vi "Nabız Ölçer.vi"() -> ()   [LabVIEW 2017]
uses:
  <vilib>/MakerHub/LINX/Public/Peripherals/Analog/Analog Read 1 Chan.vi
  <vilib>/MakerHub/LINX/Public/Peripherals/Analog/Analog Read N Chans.vi
  <vilib>/MakerHub/LINX/Private/Local IO/LinxAnalogRead.vi
  <vilib>/MakerHub/LINX/Public/Utilities/Check Channel.vi
  <vilib>/MakerHub/LINX/Public/Utilities/Open Serial.vi
  <vilib>/MakerHub/LINX/Private/Utilties/Generate Error.vi
  <vilib>/MakerHub/LINX/LMH-LINX.lvlib
panel:
  in  "Serial Port":refnum<visa-resource-name>="N/A"
  in  "Analog Channel":u8
  out "Waveform Chart":dbl(graph)
  in  "Stop":bool
  out "nabız":dbl
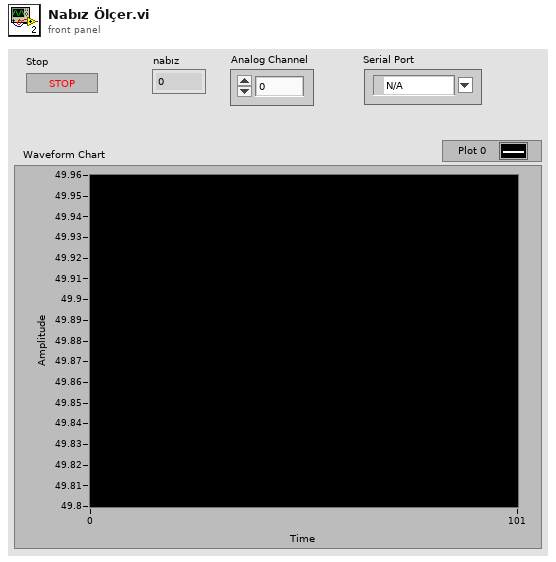
[diagram p1: front panel]
types:
  T1 = enum16{"open", "replace", "create", "open or create", "replace or create", "replace or create with confirmation"}
  T2 = typedef "LMH-LINX.lvlib/LINX Ref.ctl" = cluster{"IO":T3, "Interface":T4, "LINX Device Config":T5}
  T3 = typedef "LMH-LINX.lvlib/Platform.ctl" = enum16{"Remote", "Local"}
  T4 = typedef "LMH-LINX.lvlib/Interface.ctl" = enum16{"Serial", "TCP"}
  T5 = typedef "LMH-LINX.lvlib/Device.lvlib/LINX Device Config.ctl" = cluster{"Interface":T4, "COM Port":refnum<visa-resource-name>, "TCP Configuration":T6, "Device Family":u8, "Device ID":u8, "Device Name":string, "TCP Ref":refnum<k5>, "Channels":T7}
  T6 = typedef "LMH-LINX.lvlib/Device.lvlib/TCP Config.ctl" = cluster{"IP Address":string, "Port":u16}
  T7 = typedef "LMH-LINX.lvlib/Channels.ctl" = cluster{"DI":u8[], "DO":u8[], "AI":u8[], "AO":u8[], "PWM":u8[], "QE":u8[], "UART":u8[], "I2C 2":u8[], "SPI":u8[], "CAN":u8[], "Servo":u8[], "AI Ref (V)":dbl, "AI Resolution (Bits)":u8, "AO Ref (V)":dbl, "AO Resolution (Bits)":u8}
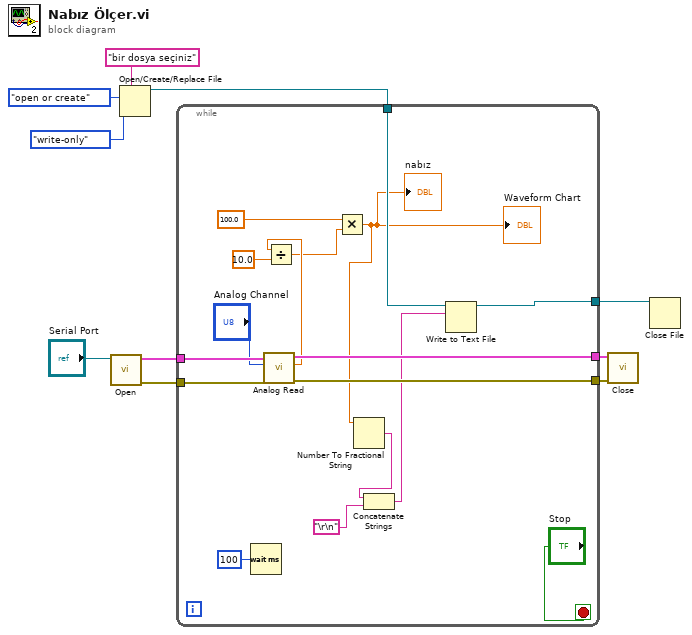
[diagram p0: block diagram]
diagram:
  n1 = call-poly <vilib>:"Open.vi"("Serial Port"="Serial Port") -> ("Error Out"=w7:errorcluster, "LINX Resource"=w8:T2)  [unwired: 8 in, 1 out]
  n2 = Open/Create/Replace File(prompt="bir dosya seçiniz", operation (0:open)=T1."open or create", access (0:read/write)=enum16{"read/write", "read-only", "write-only"}."write-only") -> (refnum out=w5:refnum<file>)  [unwired: 3 in, 2 out]
  n3 = while {
    tunnel: [w26] -> w10
    tunnel: [w25] -> w9
    tunnel: w8 -> [w24]
    tunnel: w7 -> [w23]
    tunnel: w5 -> [w22]
    tunnel: [w21] -> w4
    stop <- "Stop" stop-if-true
    n4 = Wait (ms)(milliseconds to wait=u32 100) -> ()  [unwired: 1 out]
    n5 = call-poly <vilib>:"Analog Read.vi"("Error In"=w23, "Analog Channel"="Analog Channel", "LINX Resource"=w24) -> ("Error Out"=w25:errorcluster, "Voltage"=w14:dbl, "LINX Resource"=w26:T2)  [unwired: 5 in, 1 out]
    n6 = Divide(x=w14, y=10.0) -> (x/y=w12:dbl)
    n7 = Multiply(x=100.0, y=w12) -> (x*y=w16:dbl)
    "nabız" <- w16
    "Waveform Chart" <- w16
    n8 = Number To Fractional String(number=w16) -> (F-format string=w18:string)  [unwired: 3 in]
    n9 = Concatenate Strings(w18, "\r\n") -> (w19:string)
    n10 = Write to Text File(file (use dialog)=w22, text=w19) -> (refnum out=w21:refnum<file>)  [unwired: 2 in, 2 out]
  }
  n11 = call <vilib>:"Close.vi"("Error In"=w9, "LINX Resource"=w10) -> ()  [unwired: 9 in, 1 out]
  n12 = Close File(refnum=w4) -> ()  [unwired: 1 in, 2 out]
